vi "DPT TC Panel Init.vi"(11 "TC Panel":T1[][](array[typedef])) -> (3 "TC Panel 1":T1[][](array[typedef]))   [LabVIEW 2016]
doc: "Initialize first 3 panel elements in Panel 1 to be RDB F, Room Ambient, and Tscale."
uses:
  Type Definitions/DPT Channel Label.ctl
  Utility/Custom Pallet Controls/Custom Pallet String.ctl
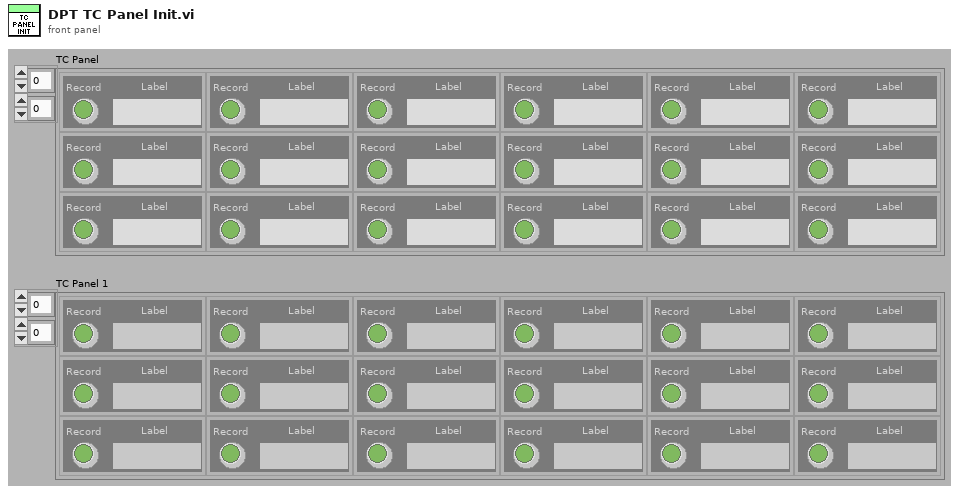
[diagram p1: front panel]
types:
  T1 = typedef "DPT Channel Label.ctl" = cluster{"Label":T2, "Record":bool, "Index":u32, "Channel":string}
  T2 = typedef "Custom Pallet String.ctl" = string
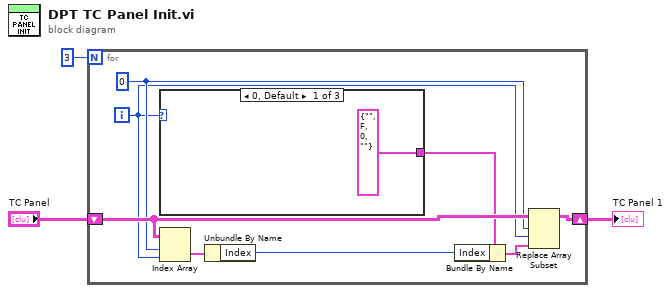
[diagram p0: block diagram]
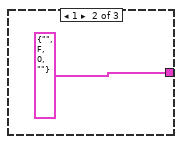
[diagram p2: hidden frame]
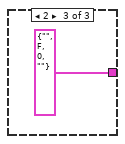
[diagram p3: hidden frame]
diagram:
  n1 = for {
    N: 3 -> [_]
    shift-right: [w11] -> w1
    shift-left: "TC Panel" -> [w10]
    i -> [w5]
    w9 = 0 ("index (row)")
    n2 = case shown="0, Default" w5 {
      tunnel: [T1 {"Label"="", "Record"=FALSE, "Index"=0, "Channel"=""} ("Sensor 2") T1 {"Label"="", "Record"=FALSE, "Index"=0, "Channel"=""} ("Sensor 2") T1 {"Label"="", "Record"=FALSE, "Index"=0, "Channel"=""} ("Sensor 2")] -> w4
      frame 0, Default {
      }
      frame 1 {
      }
      frame 2 {
      }
    }
    n3 = Index Array(array=w10, index (row)=w9, index (col)=w5) -> (element=w8:T1)
    n4 = Unbundle By Name(w8) -> ("Index"=w7:u32)
    n5 = Bundle By Name(cluster=w4, "Index"=w7) -> (w6:T1)
    n6 = Replace Array Subset(array=w10, new element=w6, index (row)=w9, index (col)=w5) -> (w11:T1[][])
  }
  "TC Panel 1" <- w1
